vi "18-Split.vi"(11 "Snailfish Number in":string) -> (2 "Split?":bool, 3 "Snailfish Number out":string)   [LabVIEW 2019, in "18.lvlib"]
uses:
  18.lvlib
  <vilib>/regexp/Match Regular Expression.xnode
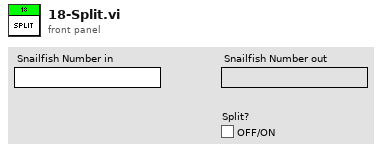
[diagram p1: front panel]
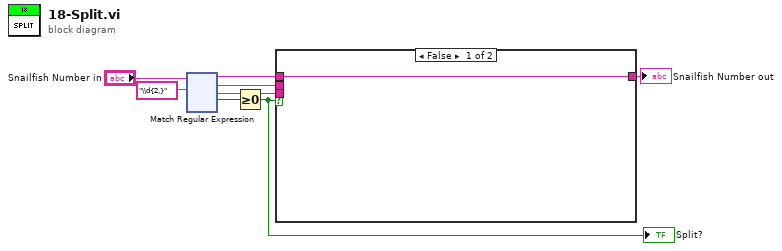
[diagram p0: block diagram]
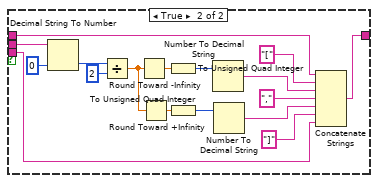
[diagram p2: hidden frame]
diagram:
  n1 = xnode "Match Regular Expression"("input string"="Snailfish Number in", "regular expression"="\\d{2,}") -> ("before match"=w4:string, "whole match"=w5:string, "after match"=w3:string, "offset past match"=w7:i32)  [unwired: 4 in, 1 out]
  n2 = Greater Or Equal To 0?(x=w7) -> (x >= 0?=w1:bool)
  "Split?" <- w1
  n3 = case shown="False" w1 {
    tunnel: w5 -> [_ w26]
    tunnel: w4 -> [w9 w12]
    tunnel: w3 -> [_ w11]
    tunnel: [w9 w10] -> w2
    frame False {
    }
    frame True {
      n4 = Decimal String To Number(string=w26, default (0L)=u64 0 ("default (0 I32)")) -> (number=w24:u64)  [unwired: 1 in, 1 out]
      n5 = Divide(x=w24, y=u64 2) -> (x/y=w22:dbl)
      n6 = Round Toward -Infinity(1:w22) -> (0:w21:dbl)
      n7 = Round Toward +Infinity(x=w22) -> (ceil(x): smallest int >= x=w19:dbl)
      n8 = To Unsigned Quad Integer(1:w21) -> (0:w20:u64)
      n9 = To Unsigned Quad Integer(1:w19) -> (0:w18:u64)
      n10 = Number To Decimal String(number=w20) -> (decimal integer string=w16:string)  [unwired: 1 in]
      n11 = Number To Decimal String(number=w18) -> (decimal integer string=w14:string)  [unwired: 1 in]
      n12 = Concatenate Strings(w12, "[", w16, "," ("string"), w14, "]" ("string"), w11) -> (w10:string)
    }
  }
  "Snailfish Number out" <- w2
